vi "TREE_Clear.vi"(8 "error in":errorcluster, 11 "Tree Ref":refnum<vi>) -> (0 "error out":errorcluster, 3 "Tree Ref":refnum<vi>)   [LabVIEW 2016]
doc: "Set a customize symbol for a item. Notice that all the symbol of items have the same symbol index will change. Set a new symbol index if you want to customize a single item."
panel:
  # "Input"
  # "Output"
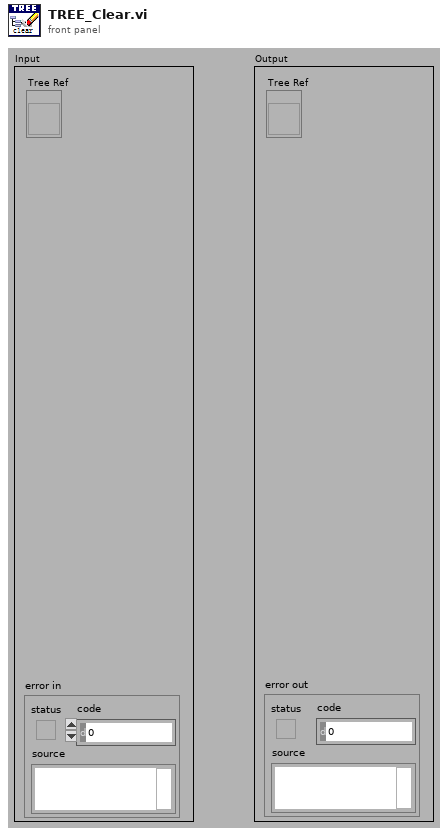
[diagram p1: front panel]
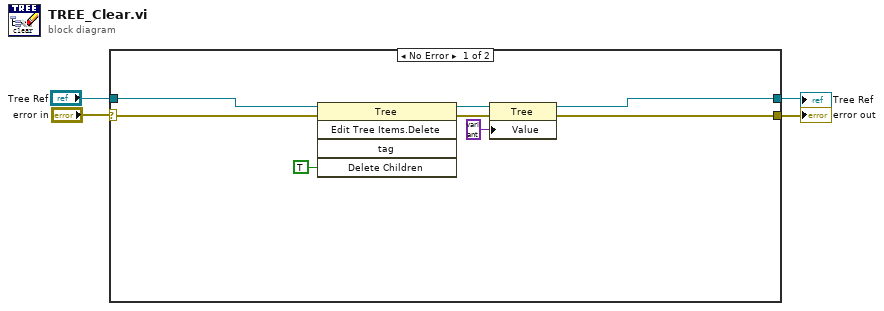
[diagram p0: block diagram]
diagram:
  n1 = case shown="No Error" "error in" {
    selector: "error in" -> [w12 w14]
    tunnel: [w5 w14] -> w4
    tunnel: [w8 w13] -> w2
    tunnel: "Tree Ref" -> [w9 w13]
    frame No Error {
      n2 = invoke class="Tree" method="Edit Tree Items.Delete"(reference=w9, error in=w12, "Delete Children"=TRUE ("删除子项？")) -> (reference out=w10:refnum<vi>, error out=w6:errorcluster)  [unwired: 2 in, 3 out]
      n3 = property class="Tree"(reference=w10, error in=w6, "Value"=variant) -> (reference out=w8:refnum<vi>, error out=w5:errorcluster)
    }
    frame Error {
    }
  }
  "error out" <- w4
  "Tree Ref" <- w2
